vi "Calculator-teardown.vi"(7 "test case ID":string, 10 "Actual result":dbl) -> (3 "result":bool)   [LabVIEW 2018]
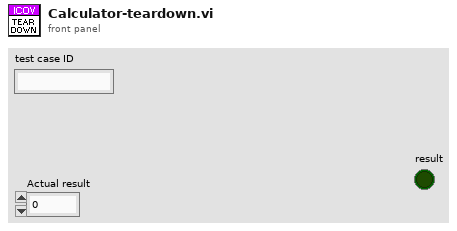
[diagram p1: front panel]
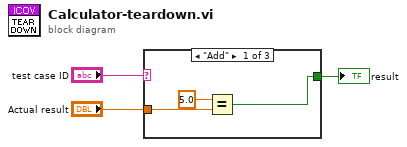
[diagram p0: block diagram]
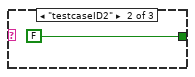
[diagram p2: hidden frame]
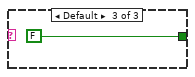
[diagram p3: hidden frame]
diagram:
  n1 = case shown="\"Add\"" "test case ID" {
    tunnel: [w4 FALSE FALSE] -> w2
    tunnel: "Actual result" -> [w6 _ _]
    frame "Add" {
      n2 = Equal?(x=5.0, y=w6) -> (x = y?=w4:bool)
    }
    frame "testcaseID2" {
    }
    frame Default {
    }
  }
  "result" <- w2
